vi "Main.vi"() -> ()   [LabVIEW 2017]
doc: "The myRIO Project template acquires acceleration data from the onboard accelerometer and displays the changes of acceleration values in a waveform chart."
uses:
  Y Axis Motor Cluster.ctl
  X Axis Motor Cluster.ctl
  Coords Input Cluster.ctl
  Motor Status Enum.ctl
  Encoder Cluster.ctl
  <vilib>/myRIO/Common/Instrument Driver Framework/myRIO v1.0/Encoder/typedefs/Encoder Count Direction Enum.ctl
  Motion Type Def.ctl
  <vilib>/myRIO/Instrument Drivers/Onboard IO/PWM/typedefs/PWM Reference.ctl
  <vilib>/myRIO/Common/Instrument Driver Framework/Utilities/typedefs/myRIO Generic Hardware Reference.ctl
  <vilib>/myRIO/Common/Instrument Driver Framework/Utilities/typedefs/Hardware Version Enum.ctl
  <vilib>/myRIO/Common/Instrument Driver Framework/Utilities/typedefs/myRIO v1.0 Reference.ctl
  <vilib>/myRIO/Common/Instrument Driver Framework/Utilities/typedefs/Generic FPGA Reference.ctl
  <vilib>/myRIO/Common/Instrument Driver Framework/myRIO v1.0/PWM/typedefs/PWM Channels Enum.ctl
  <vilib>/myRIO/Instrument Drivers/Onboard IO/PWM/typedefs/PWM Configuration.ctl
  <vilib>/userdefined/High Color/nirio_resource_hc.ctl
  <vilib>/myRIO/Common/Instrument Driver Framework/Utilities/vis/Is FPGA Ref Available.vi
  <vilib>/myRIO/Common/Instrument Driver Framework/myRIO v1.0/PWM/vis/myRIO v1.1 Open PWM.vi
  <vilib>/myRIO/Instrument Drivers/Onboard IO/PWM/vis/Set Duty Cycle and Frequency.vi
  <vilib>/myRIO/Common/Instrument Driver Framework/Utilities/vis/Validate Channels.vi
  <vilib>/myRIO/Common/Instrument Driver Framework/myRIO v1.0/PWM/vis/myRIO v1.0 Reserve PWM.vi
  <vilib>/myRIO/Common/Instrument Driver Framework/myRIO v1.0/UART/vis/myRIO v1.0 Close UART.vi
  <vilib>/myRIO/Common/Instrument Driver Framework/myRIO v1.0/PWM/vis/myRIO v1.0 Build MUX Configuration PWM.vi
  <vilib>/myRIO/Common/Instrument Driver Framework/myRIO v1.0/Resource Manager/vis/myRIO v1.0 Reserve Channel List.vi
  <vilib>/myRIO/Common/Instrument Driver Framework/myRIO v1.0/Resource Manager/vis/myRIO v1.0 Create Configuration List.vi
  <vilib>/myRIO/Common/Instrument Driver Framework/myRIO v1.0/Resource Manager/vis/myRIO v1.0 Reserve Channel.vi
  <vilib>/myRIO/Common/Instrument Driver Framework/myRIO v1.0/Resource Manager/vis/myRIO v1.0 Unreserve Channel.vi
  <vilib>/myRIO/Common/Instrument Driver Framework/myRIO v1.0/Resource Manager/vis/myRIO v1.0 Build Mutex Name.vi
  <vilib>/Utility/VariantDataType/GetNumericInfo.vi
  <vilib>/Utility/error.llb/Error Cluster From Error Code.vi
  <vilib>/myRIO/Common/Instrument Driver Framework/myRIO v1.0/myRIO v1.1 Open.vi
  <vilib>/myRIO/Common/Instrument Driver Framework/Utilities/vis/IO Manager.vi
  <vilib>/myRIO/Common/Instrument Driver Framework/Utilities/vis/Configuration Manager.vi
  <vilib>/myRIO/Common/Instrument Driver Framework/myRIO v1.0/Resource Manager/vis/myRIO v1.0 Configure IO.vi
  <vilib>/myRIO/Common/Instrument Driver Framework/myRIO v1.0/myRIO v1.0 Close.vi
  <vilib>/myRIO/Common/Instrument Driver Framework/myRIO v1.0/PWM/vis/myRIO v1.0 Write PWM.vi
  <vilib>/myRIO/Common/Instrument Driver Framework/Utilities/vis/FPGA Ref Manager.vi
  <vilib>/myRIO/Common/Instrument Driver Framework/myRIO v1.0/myRIO v1.0 Reset FPGA.vi
  <vilib>/myRIO/Common/Instrument Driver Framework/myRIO v1.0/IRQ/vis/myRIO v1.0 IRQ Info FGV.vi
  <vilib>/myRIO/Common/Instrument Driver Framework/myRIO v1.0/IRQ/vis/myRIO v1.0 Timer IRQ Info FGV.vi
  <vilib>/myRIO/Common/Instrument Driver Framework/myRIO v1.0/IRQ/vis/myRIO v1.0 ISR Agent.vi
  <vilib>/myRIO/Express VI/Onboard IO/PWM/PWM Express VI.xnode
  <vilib>/myRIO/Instrument Drivers/Onboard IO/PWM/vis/myRIO PWM Open.xnode
  <vilib>/myRIO/Instrument Drivers/Utilities/Utilities.lvlib
  <vilib>/myRIO/Instrument Drivers/Onboard IO/PWM/PWM.lvlib
panel:
  out "Converted Decel":dbl
  out "Converted Accel":dbl
  out "Motion Profile":T1=enum."Triangular"
  out "Converted\nPWM Freq":dbl
  in  "Y Axis Setpoint":T2
  out "X Axis 2":T3(graph)
  out "Y Axis 2":T3(graph)
  out "Encoder Output":T4
  out "X Axis state":T6
  out "Y Axis state":T6
  out "Loop Runtime (s)":dbl format="%.3f"
  in  "Clear Chart History":bool
  in  "Coordinates Input":T7
  out "Y Axis":T8(graph)
  out "X Axis":T8(graph)
  in  "X Axis Motor Target":T9
  out "X Axis Motor Params":T10
  out "Y Axis Motor Params":T11
  in  "stop":bool
  out "Total Runtime (s)":dbl format="%.2f"
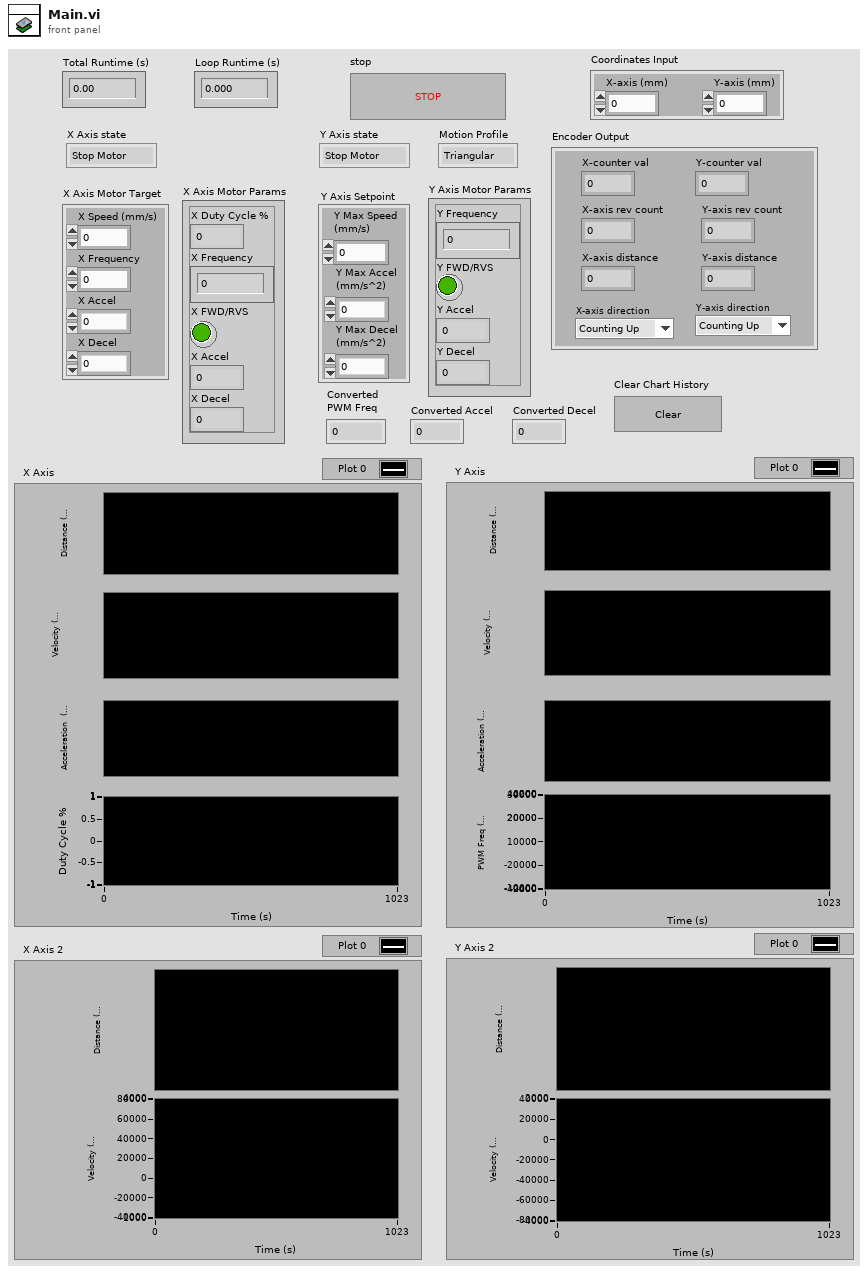
[diagram p1: front panel]
types:
  T1 = typedef "Motion Type Def.ctl" = enum16{"Trapezodial", "Triangular"}
  T2 = cluster{"Y Max Speed \n(mm/s)":dbl, "Y Max Accel\n(mm/s^2)":dbl, "Y Max Decel \n(mm/s^2)":dbl}
  T3 = cluster{"Velocity (mm/s)":dbl, "Acceleration (mm/s^2)":dbl}
  T4 = typedef "Encoder Cluster.ctl" = cluster{"Y-axis rev count":dbl, "Y-axis distance":dbl, "X-axis rev count":dbl, "X-axis distance":dbl, "Y-axis direction":T5, "X-axis direction":T5, "X-counter val":i32, "Y-counter val":i32}
  T5 = typedef "Encoder Count Direction Enum.ctl" = enum16{"Counting Up", "Counting Down"}
  T6 = typedef "Motor Status Enum.ctl" = enum16{"Stop Motor", "Read Inputs", "Steady Speed", "Accelerate", "Decelerate"}
  T7 = typedef "Coords Input Cluster.ctl" = cluster{"X-axis (mm)":dbl, "Y-axis (mm)":dbl}
  T8 = cluster{"X-axis distance":dbl, dbl, dbl, "X Frequency":dbl}
  T9 = cluster{"X Frequency":dbl, "X Accel":dbl, "X Decel":dbl, "X Speed (mm/s)":dbl}
  T10 = typedef "X Axis Motor Cluster.ctl" = cluster{"X Frequency":dbl, "X FWD/RVS":bool, "X Accel":dbl, "X Decel":dbl, "X Duty Cycle %":dbl}
  T11 = typedef "Y Axis Motor Cluster.ctl" = cluster{"Y Frequency":dbl, "Y FWD/RVS":bool, "Y Accel":dbl, "Y Decel":dbl}
  T12 = cluster{"X Frequency":dbl, "X FWD/RVS":bool, "X Accel":dbl, "X Decel":dbl, "X Duty Cycle %":dbl}
  T13 = cluster{"Y Frequency":dbl, "Y FWD/RVS":bool, "Y Accel":dbl, "Y Decel":dbl}
  T14 = cluster{"X-axis distance":dbl, dbl, dbl, "X Frequency":dbl}[]
  T15 = cluster{" Distance target (mm)":dbl, "Max Accel (mm/s^2)":dbl, "Max Decel (mm/s^2)":dbl, "Velocity Limit (mm/s) ":dbl, "Time step (s)":dbl}
  T16 = enum16{"800", "1600", "3200", "6400", "12800", "25600"}
  T17 = cluster{"Cruising Speed (mm/s)":dbl, "Crusing Time (s)":dbl, "Decel Time (s)":dbl, "Accel Time (s)":dbl, "Total Time (s)":dbl, "Accel Distance (mm)":dbl, "Decel Distance (mm)":dbl, "Crusing Distance (mm)":dbl}
  T18 = cluster{"Y-axis distance":dbl, dbl, dbl, "Y Frequency":dbl}
  T19 = cluster{"X-axis rev count":dbl, dbl, dbl, "X Duty Cycle %":dbl}
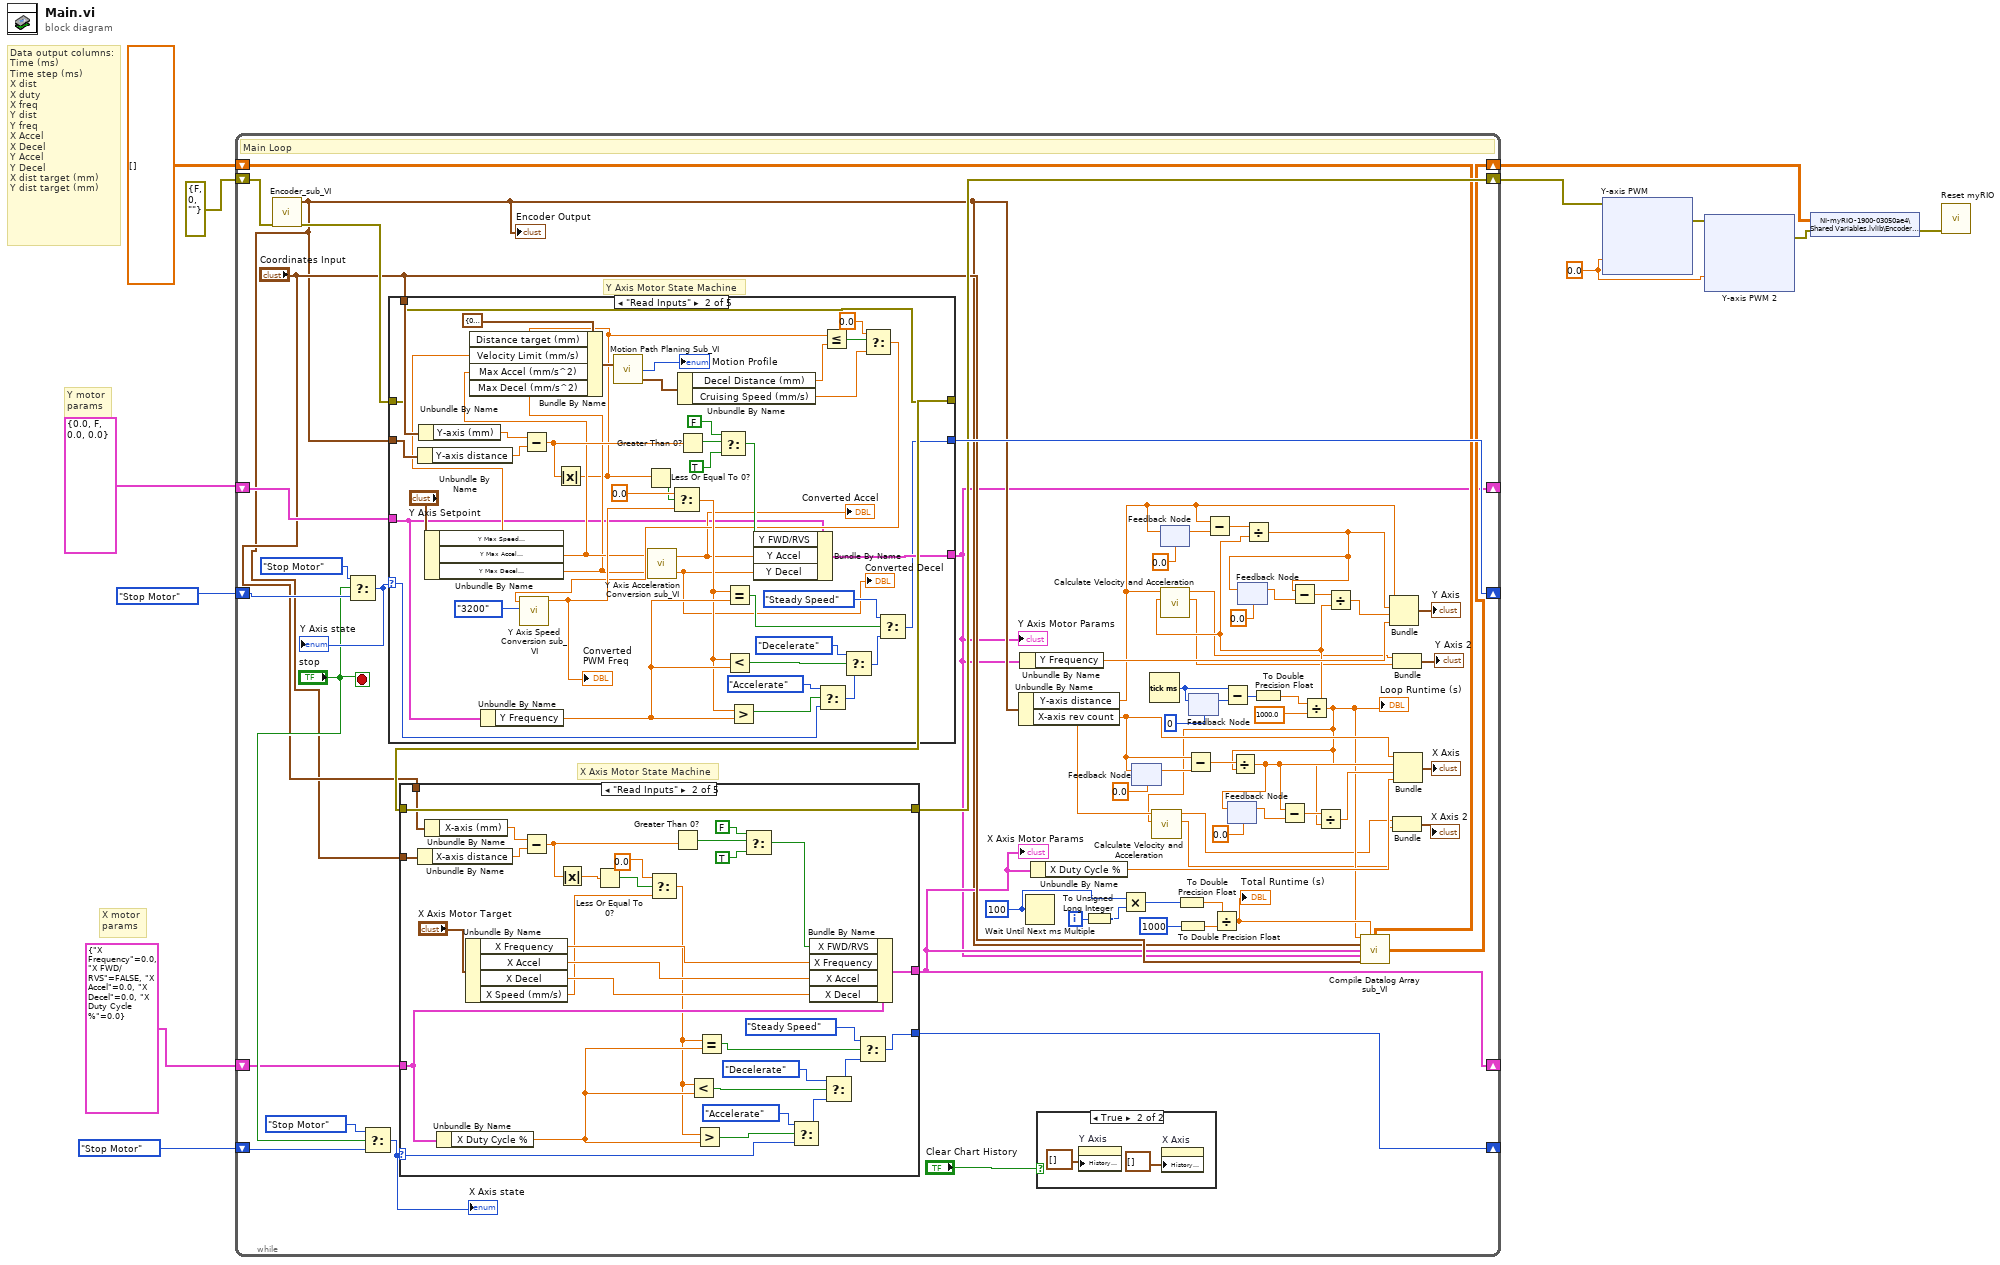
[diagram p0: block diagram]
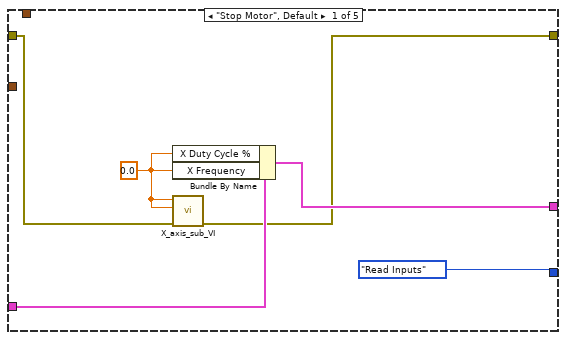
[diagram p3: hidden frame]
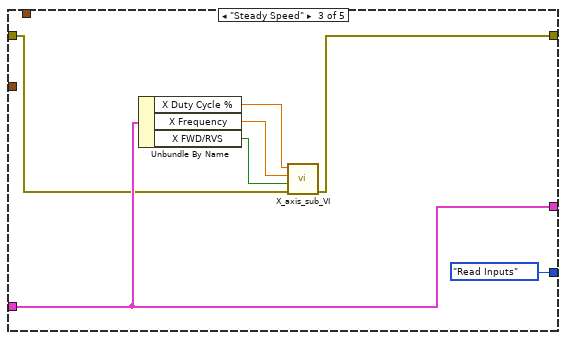
[diagram p4: hidden frame]
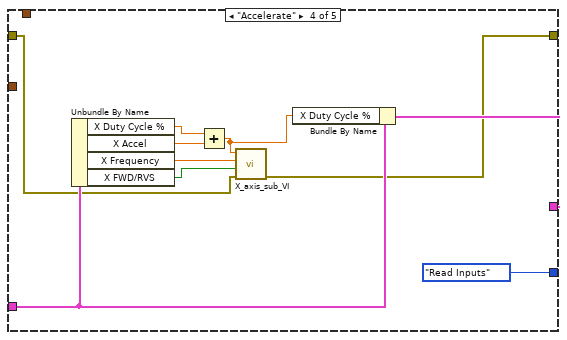
[diagram p5: hidden frame]
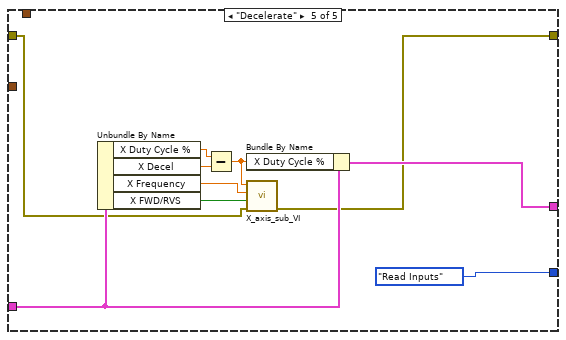
[diagram p6: hidden frame]
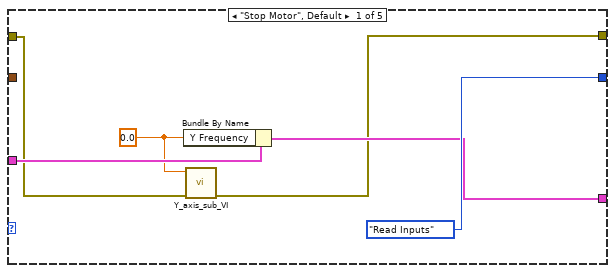
[diagram p7: hidden frame]
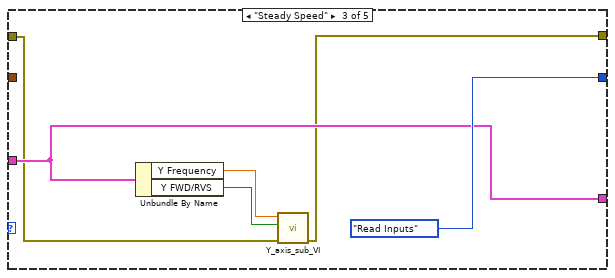
[diagram p8: hidden frame]
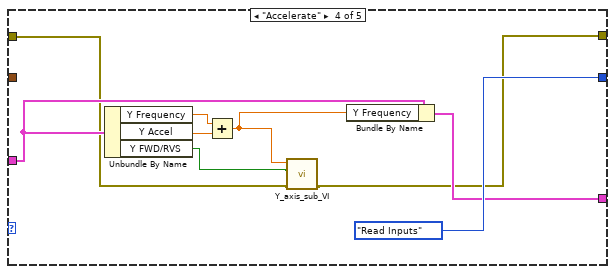
[diagram p9: hidden frame]
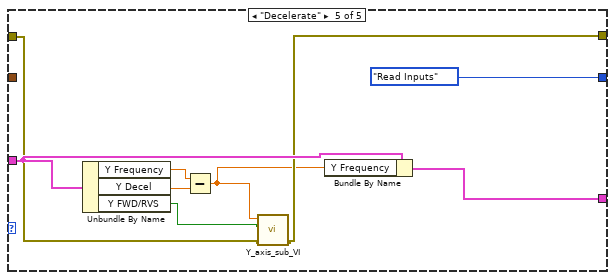
[diagram p10: hidden frame]
diagram:
  w6 = 0.0 ("Frequency [Hz]")
  # "X motor \nparams"
  # "Y motor \nparams"
  # "Data output columns:\nTime (ms)\nTime step (ms)\nX dist\nX duty\nX freq\nY dist\nY freq\nX Accel\nX Decel\nY Accel\nY Decel\nX dist target (mm)\nY dist target (mm)"
  n1 = while {
    shift-right: [w63] -> w12
    shift-left: errorcluster {"status"=FALSE, "code"=0, "source"=""} ("error in (no error)") -> [w77]
    shift-right: [w45] -> w1
    shift-left: dbl[][] [] -> [w46]
    shift-right: [w38] -> _
    shift-left: T13 {"Y Frequency"=0.0, "Y FWD/RVS"=FALSE, "Y Accel"=0.0, "Y Decel"=0.0} ("Y Axis Motor Params 2") -> [w76]
    shift-right: [w75] -> _
    shift-left: Motor_Status_Enum."Stop Motor" -> [w73]
    shift-right: [w66] -> _
    shift-left: Motor_Status_Enum."Stop Motor" -> [w68]
    shift-right: [w42] -> _
    shift-left: T12 {"X Frequency"=0.0, "X FWD/RVS"=FALSE, "X Accel"=0.0, "X Decel"=0.0, "X Duty Cycle %"=0.0} ("X Axis Motor Params 3") -> [w65]
    i -> [w52]
    stop <- "stop" stop-if-true
    w51 = u32 100 ("milliseconds to wait")
    # "X Axis Motor State Machine"
    # "Y Axis Motor State Machine"
    # "Main Loop"
    n2 = call "Encoder_sub_VI.vi"("error in (no error)"=w77) -> ("error out"=w71:errorcluster, "Encoder Output"=w39:T4)  [unwired: 9 in]
    "Encoder Output" <- w39
    n3 = Select(t=Motor_Status_Enum."Stop Motor", s="stop", f=w73) -> (s? t:f=w74:T6)
    "Y Axis state" <- w74
    n4 = Select(t=Motor_Status_Enum."Stop Motor", s="stop", f=w68) -> (s? t:f=w69:T6)
    "X Axis state" <- w69
    n5 = case shown="\"Read Inputs\"" w74 {
      selector: w74 -> [_ w152 _ _ _]
      tunnel: w76 -> [w150 w153 w197 w206 w214]
      tunnel: [Motor_Status_Enum."Read Inputs" w151 Motor_Status_Enum."Read Inputs" Motor_Status_Enum."Read Inputs" Motor_Status_Enum."Read Inputs"] -> w75
      tunnel: [w148 w158 w197 w205 w215] -> w38
      tunnel: w71 -> [w146 w155 w196 w202 w212]
      tunnel: [w147 w155 w195 w201 w213] -> w64
      tunnel: w39 -> [_ w157 _ _ _]
      tunnel: "Coordinates Input" -> [_ w156 _ _ _]
      frame "Stop Motor", Default {
        w145 = 0.0 ("Y Frequency")
        n6 = Bundle By Name(cluster=w150, "Y Frequency"=w145) -> (w148:T13)
        n7 = call "Y_axis_sub_VI.vi"("error in (no error)"=w146, "Frequency"=w145) -> ("error out"=w147:errorcluster)  [unwired: 9 in]
      }
      frame "Read Inputs" {
        n8 = Unbundle By Name(w157) -> ("Y-axis distance"=w175:dbl)
        n9 = Unbundle By Name(w156) -> ("Y-axis (mm)"=w176:dbl)
        n10 = Unbundle By Name("Y Axis Setpoint") -> ("Y Max Speed \n(mm/s)"=w154:dbl, "Y Max Accel\n(mm/s^2)"=w161:dbl, "Y Max Decel \n(mm/s^2)"=w160:dbl)
        n11 = Unbundle By Name(w153) -> ("Y Frequency"=w190:dbl)
        n12 = Subtract(x=w176, y=w175) -> (x-y=w170:dbl)
        n13 = Absolute Value(x=w170) -> (abs(x)=w159:dbl)
        n14 = Bundle By Name(cluster=T15 {" Distance target (mm)"=0.0, "Max Accel (mm/s^2)"=0.0, "Max Decel (mm/s^2)"=0.0, "Velocity Limit (mm/s) "=0.0, "Time step (s)"=0.0} ("Motion Planning Inputs"), "Distance target (mm)"=w159, "Velocity Limit (mm/s)"=w154, "Max Accel (mm/s^2)"=w161, "Max Decel (mm/s^2)"=w160) -> (w173:T15)
        n15 = call "Motion Path Planing Sub_VI.vi"("Motion Planning Inputs"=w173) -> ("Motion Profile"=→"Motion Profile":T1, "Motion Planning Outputs"=w171:T17)  [unwired: 4 in, 1 out]
        n16 = Less Or Equal To 0?(x=w159) -> (x <= 0?=w174:bool)
        n17 = call "Y Axis Acceleration Conversion sub_VI.vi"("Deceleration (mm/s^2)"=w160, "Acceleration (mm/s^2)"=w161) -> ("Freq decrease per 0.1ms (Hz)"=w162:dbl, "Freq increase per 0.1ms (Hz)"=w163:dbl)
        "Converted Accel" <- w163
        "Converted Decel" <- w162
        n18 = Unbundle By Name(w171) -> ("Decel Distance (mm)"=w169:dbl, "Cruising Speed (mm/s)"=w165:dbl)
        n19 = Greater Than 0?(x=w170) -> (x > 0?=w181:bool)
        n20 = Select(t=FALSE, s=w181, f=TRUE) -> (s? t:f=w182:bool)
        n21 = Bundle By Name(cluster=w153, "Y FWD/RVS"=w182, "Y Accel"=w163, "Y Decel"=w162) -> (w158:T13)
        n22 = Less Or Equal?(x=w159, y=w169) -> (x <= y?=w168:bool)
        n23 = Select(t=0.0, s=w168, f=w165) -> (s? t:f=w166:dbl)
        n24 = call "Y Axis Speed Conversion sub_VI.vi"("Microsteps per Rev"=T16."3200", "Setpoint\nSpeed (mm/s)"=w166) -> ("PWM Frequency"=w178:dbl)  [unwired: 9 in]
        "Converted\nPWM Freq" <- w178
        n25 = Select(t=0.0, s=w174, f=w178) -> (s? t:f=w179:dbl)
        n26 = Equal?(x=w179, y=w190) -> (x = y?=w191:bool)
        n27 = Less?(x=w179, y=w190) -> (x < y?=w187:bool)
        n28 = Greater?(x=w179, y=w190) -> (0:w194:bool)
        n29 = Select(t=Motor_Status_Enum."Accelerate", s=w194, f=w152) -> (s? t:f=w189:T6)
        n30 = Select(t=Motor_Status_Enum."Decelerate", s=w187, f=w189) -> (s? t:f=w192:T6)
        n31 = Select(t=Motor_Status_Enum."Steady Speed", s=w191, f=w192) -> (s? t:f=w151:T6)
      }
      frame "Steady Speed" {
        n32 = Unbundle By Name(w197) -> ("Y Frequency"=w199:dbl, "Y FWD/RVS"=w200:bool)
        n33 = call "Y_axis_sub_VI.vi"("error in (no error)"=w196, "FWD/RVS"=w200, "Frequency"=w199) -> ("error out"=w195:errorcluster)  [unwired: 8 in]
      }
      frame "Accelerate" {
        n34 = Unbundle By Name(w206) -> ("Y Frequency"=w208:dbl, "Y Accel"=w209:dbl, "Y FWD/RVS"=w203:bool)
        n35 = Add(x=w208, y=w209) -> (x+y=w204:dbl)
        n36 = call "Y_axis_sub_VI.vi"("error in (no error)"=w202, "FWD/RVS"=w203, "Frequency"=w204) -> ("error out"=w201:errorcluster)  [unwired: 8 in]
        n37 = Bundle By Name(cluster=w206, "Y Frequency"=w204) -> (w205:T13)
      }
      frame "Decelerate" {
        n38 = Unbundle By Name(w214) -> ("Y Frequency"=w218:dbl, "Y Decel"=w217:dbl, "Y FWD/RVS"=w211:bool)
        n39 = Subtract(x=w218, y=w217) -> (x-y=w210:dbl)
        n40 = call "Y_axis_sub_VI.vi"("error in (no error)"=w212, "FWD/RVS"=w211, "Frequency"=w210) -> ("error out"=w213:errorcluster)  [unwired: 8 in]
        n41 = Bundle By Name(cluster=w214, "Y Frequency"=w210) -> (w215:T13)
      }
    }
    "Y Axis Motor Params" <- w38
    n42 = case shown="\"Read Inputs\"" w69 {
      selector: w69 -> [_ w105 _ _ _]
      tunnel: [Motor_Status_Enum."Read Inputs" w98 Motor_Status_Enum."Read Inputs" Motor_Status_Enum."Read Inputs" Motor_Status_Enum."Read Inputs"] -> w66
      tunnel: [w82 w104 w121 w128 w138] -> w42
      tunnel: w65 -> [w83 w103 w121 w127 w137]
      tunnel: w64 -> [w81 w101 w119 w126 w136]
      tunnel: [w80 w101 w118 w125 w135] -> w63
      tunnel: w39 -> [_ w100 _ _ _]
      tunnel: "Coordinates Input" -> [_ w99 _ _ _]
      frame "Stop Motor", Default {
        w85 = 0.0 ("Y Frequency")
        n43 = Bundle By Name(cluster=w83, "X Duty Cycle %"=w85, "X Frequency"=w85) -> (w82:T12)
        n44 = call "X_axis_sub_VI.vi"("error in (no error)"=w81, "Frequency"=w85, "Duty Cycle %"=w85) -> ("error out"=w80:errorcluster)  [unwired: 8 in]
      }
      frame "Read Inputs" {
        n45 = Unbundle By Name(w100) -> ("X-axis distance"=w89:dbl)
        n46 = Unbundle By Name(w99) -> ("X-axis (mm)"=w90:dbl)
        n47 = Unbundle By Name(w103) -> ("X Duty Cycle %"=w116:dbl)
        n48 = Unbundle By Name("X Axis Motor Target") -> ("X Frequency"=w108:dbl, "X Accel"=w106:dbl, "X Decel"=w107:dbl, "X Speed (mm/s)"=w94:dbl)
        n49 = Subtract(x=w90, y=w89) -> (x-y=w86:dbl)
        n50 = Absolute Value(x=w86) -> (abs(x)=w87:dbl)
        n51 = Less Or Equal To 0?(x=w87) -> (x <= 0?=w88:bool)
        n52 = Select(t=0.0, s=w88, f=w94) -> (s? t:f=w93:dbl)
        n53 = Greater Than 0?(x=w86) -> (x > 0?=w96:bool)
        n54 = Less?(x=w93, y=w116) -> (x < y?=w111:bool)
        n55 = Greater?(x=w93, y=w116) -> (0:w109:bool)
        n56 = Equal?(x=w93, y=w116) -> (x = y?=w115:bool)
        n57 = Select(t=FALSE, s=w96, f=TRUE) -> (s? t:f=w91:bool)
        n58 = Select(t=Motor_Status_Enum."Accelerate", s=w109, f=w105) -> (s? t:f=w113:T6)
        n59 = Bundle By Name(cluster=w103, "X FWD/RVS"=w91, "X Frequency"=w108, "X Accel"=w106, "X Decel"=w107) -> (w104:T12)
        n60 = Select(t=Motor_Status_Enum."Decelerate", s=w111, f=w113) -> (s? t:f=w114:T6)
        n61 = Select(t=Motor_Status_Enum."Steady Speed", s=w115, f=w114) -> (s? t:f=w98:T6)
      }
      frame "Steady Speed" {
        n62 = Unbundle By Name(w121) -> ("X Duty Cycle %"=w123:dbl, "X Frequency"=w122:dbl, "X FWD/RVS"=w124:bool)
        n63 = call "X_axis_sub_VI.vi"("error in (no error)"=w119, "FWD/RVS"=w124, "Frequency"=w122, "Duty Cycle %"=w123) -> ("error out"=w118:errorcluster)  [unwired: 7 in]
      }
      frame "Accelerate" {
        n64 = Unbundle By Name(w127) -> ("X Duty Cycle %"=w130:dbl, "X Accel"=w131:dbl, "X Frequency"=w132:dbl, "X FWD/RVS"=w134:bool)
        n65 = Add(x=w130, y=w131) -> (x+y=w133:dbl)
        n66 = call "X_axis_sub_VI.vi"("error in (no error)"=w126, "FWD/RVS"=w134, "Frequency"=w132, "Duty Cycle %"=w133) -> ("error out"=w125:errorcluster)  [unwired: 7 in]
        n67 = Bundle By Name(cluster=w127, "X Duty Cycle %"=w133) -> (w128:T12)
      }
      frame "Decelerate" {
        n68 = Unbundle By Name(w137) -> ("X Duty Cycle %"=w140:dbl, "X Decel"=w141:dbl, "X Frequency"=w142:dbl, "X FWD/RVS"=w144:bool)
        n69 = Subtract(x=w140, y=w141) -> (x-y=w143:dbl)
        n70 = Bundle By Name(cluster=w137, "X Duty Cycle %"=w143) -> (w138:T12)
        n71 = call "X_axis_sub_VI.vi"("error in (no error)"=w136, "FWD/RVS"=w144, "Frequency"=w142, "Duty Cycle %"=w143) -> ("error out"=w135:errorcluster)  [unwired: 7 in]
      }
    }
    "X Axis Motor Params" <- w42
    n72 = Unbundle By Name(w39) -> ("Y-axis distance"=w21:dbl, "X-axis rev count"=w20:dbl)
    n73 = Unbundle By Name(w38) -> ("Y Frequency"=w40:dbl)
    n74 = Wait Until Next ms Multiple(millisecond multiple=w51) -> ()  [unwired: 1 out]
    n75 = Unbundle By Name(w42) -> ("X Duty Cycle %"=w41:dbl)
    n76 = case shown="True" "Clear Chart History" {
      frame False {
      }
      frame True {
        n77 = property on="Y Axis" class="WFChart (strict)"("History Data"=T14 []) -> ()  [unwired: 2 in, 2 out]
        n78 = property on="X Axis" class="WFChart (strict)"("History Data"=T14 []) -> ()  [unwired: 2 in, 2 out]
      }
    }
    n79 = To Unsigned Long Integer(number=w52) -> (unsigned 32bit integer=w50:u32)
    n80 = Multiply(x=w51, y=w50) -> (x*y=w49:u32)
    n81 = feedback #1(0.0) -> (w28:dbl)
    n82 = feedback-in #1(w20) -> ()
    n83 = Tick Count (ms)() -> (millisecond timer value=w55:u32)
    n84 = feedback #2(0.0) -> (w36:dbl)
    n85 = feedback-in #2(w21) -> ()
    n86 = To Double Precision Float(number=w49) -> (double precision float=w48:dbl)
    n87 = To Double Precision Float(number=u32 1000 ("y")) -> (double precision float=w47:dbl)
    n88 = Subtract(x=w20, y=w28) -> (x-y=w27:dbl)
    n89 = feedback-in #3(w55) -> ()
    n90 = feedback #3(u32 0) -> (w54:u32)
    n91 = Subtract(x=w21, y=w36) -> (x-y=w35:dbl)
    n92 = Divide(x=w48, y=w47) -> (x/y=w43:dbl)
    "Total Runtime (s)" <- w43
    n93 = Subtract(x=w55, y=w54) -> (x-y=w58:u32)
    n94 = feedback #4(0.0) -> (w25:dbl)
    n95 = feedback #5(0.0) -> (w33:dbl)
    n96 = To Double Precision Float(number=w58) -> (double precision float=w56:dbl)
    n97 = Divide(x=w56, y=1000.0) -> (x/y=w19:dbl)
    "Loop Runtime (s)" <- w19
    n98 = call "Calculate Velocity and Acceleration.vi"("Loop Runtime (s)"=w19, "Displacement (mm)"=w20) -> ("Acceleration (mm/s^2)"=w13:dbl, "Velocity (mm/s)"=w14:dbl)  [unwired: 8 in]
    n99 = call "Calculate Velocity and Acceleration.vi"("Loop Runtime (s)"=w19, "Displacement (mm)"=w21) -> ("Acceleration (mm/s^2)"=w16:dbl, "Velocity (mm/s)"=w17:dbl)  [unwired: 8 in]
    n100 = Divide(x=w27, y=w19) -> (x/y=w23:dbl)
    n101 = feedback-in #4(w23) -> ()
    n102 = Divide(x=w35, y=w19) -> (x/y=w32:dbl)
    n103 = feedback-in #5(w32) -> ()
    n104 = Subtract(x=w23, y=w25) -> (x-y=w24:dbl)
    n105 = Subtract(x=w32, y=w33) -> (x-y=w31:dbl)
    n106 = Divide(x=w24, y=w19) -> (x/y=w22:dbl)
    n107 = Divide(x=w31, y=w19) -> (x/y=w30:dbl)
    n108 = call "Compile Datalog Array sub_VI.vi"("Loop Runtime (s)"=w19, "Total Runtime (s)"=w43, "Initialised Array"=w46, "Encoder Output"=w39, "X Axis Motor Params"=w42, "Y Axis Motor Params"=w38, "Coordinates Input"="Coordinates Input") -> ("Data Array"=w45:dbl[][])  [unwired: 8 in]
    n109 = Bundle("Y-axis distance"=w21, w32, w30, "Y Frequency"=w40) -> (→"Y Axis":T18)  [unwired: 1 in]
    n110 = Bundle("Velocity (mm/s)"=w17, "Acceleration (mm/s^2)"=w16) -> (→"Y Axis 2":T3)  [unwired: 1 in]
    n111 = Bundle("Velocity (mm/s)"=w14, "Acceleration (mm/s^2)"=w13) -> (→"X Axis 2":T3)  [unwired: 1 in]
    n112 = Bundle("X-axis rev count"=w20, w23, w22, "X Duty Cycle %"=w41) -> (→"X Axis":T19)  [unwired: 1 in]
  }
  n113 = xnode "Y-axis PWM"("Frequency [Hz]"=w6, "error in (no error)"=w12) -> ("error out"=w8:errorcluster)
  n114 = xnode "Y-axis PWM 2"("Frequency [Hz]"=w6, "error in (no error)"=w8) -> ("error out"=w7:errorcluster)
  n115 = shared-variable "NI-myRIO-1900-03050ae4\\Shared Variables.lvlib\\Encoder Data"(w1, error in=w7) -> (error out=w9:errorcluster)
  n116 = call <vilib>:"Reset myRIO.vi"("error in (no error)"=w9) -> ()  [unwired: 10 in, 1 out]
